vi "Stop.vi"(8 "error in (no error)":errorcluster, 11 "Electrophysiology in":refnum<class "Electrophysiology.lvclass">) -> (0 "error out":errorcluster, 3 "Electrophysiology out":refnum<class "Electrophysiology.lvclass">)   [LabVIEW 2010, in "Electrophysiology.lvclass"]
uses:
  Electrophysiology.lvclass
  Electrophysiology.lvclass/Electrophysiology.ctl
  libraries/HDF5Tools/LabView/HDF5Tools.lvlib
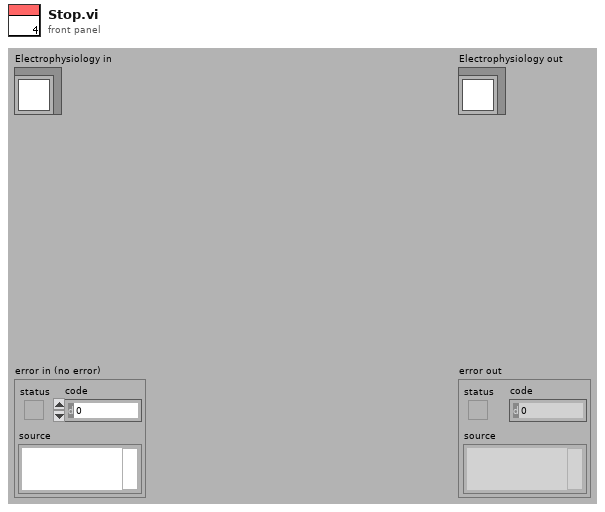
[diagram p1: front panel]
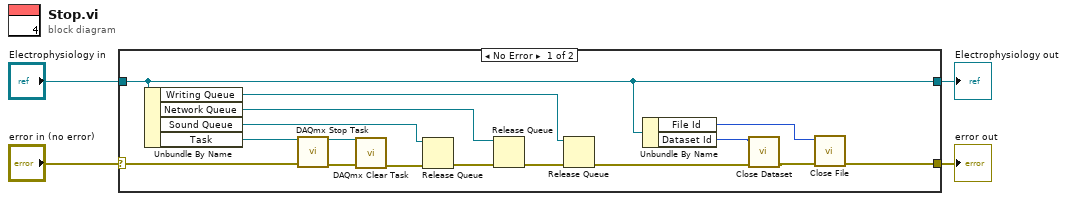
[diagram p0: block diagram]
diagram:
  n1 = case shown="No Error" "error in (no error)" {
    selector: "error in (no error)" -> [w13 w22]
    tunnel: [w5 w22] -> w3
    tunnel: [w10 w21] -> w1
    tunnel: "Electrophysiology in" -> [w10 w21]
    frame No Error {
      n2 = Unbundle By Name(w10) -> ("Writing Queue"=w11:refnum<queue>, "Network Queue"=w16:refnum<queue>, "Sound Queue"=w18:refnum<queue>, "Task"=w17:refnum<k21>)
      n3 = call <vilib>:"DAQmx Stop Task.vi"("task/channels in"=w17, "error in"=w13) -> ("task out"=w20:refnum<k21>, "error out"=w19:errorcluster)  [unwired: 12 in]
      n4 = call <vilib>:"DAQmx Clear Task.vi"("task in"=w20, "error in"=w19) -> ("error out"=w14:errorcluster)  [unwired: 13 in]
      n5 = Release Queue(queue=w18, error in (no error)=w14) -> (error out=w15:errorcluster)  [unwired: 1 in, 2 out]
      n6 = Release Queue(queue=w16, error in (no error)=w15) -> (error out=w12:errorcluster)  [unwired: 1 in, 2 out]
      n7 = Release Queue(queue=w11, error in (no error)=w12) -> (error out=w6:errorcluster)  [unwired: 1 in, 2 out]
      n8 = Unbundle By Name(w10) -> ("File Id"=w9:u64, "Dataset Id"=w8:u64)
      n9 = call "Close Dataset.vi"("error in (no error)"=w6, "dataset_id"=w8) -> ("error out"=w7:errorcluster)  [unwired: 9 in]
      n10 = call "Close File.vi"("error in (no error)"=w7, "file_id"=w9) -> ("error out"=w5:errorcluster)  [unwired: 9 in]
    }
    frame Error {
    }
  }
  "error out" <- w3
  "Electrophysiology out" <- w1
